vi "di_continuous_full.vi"() -> ()   [LabVIEW 2020]
uses:
  <vilib>/Waveform/DWDTOps.llb/DWDT Analog to Digital.vi
panel:
  out "DiFifoResidual":i32
  out "Rounds":i32
  in  "停止":bool
  out "error out":errorcluster caption="错误输出"
  out "数字波形图":digitalwaveform(graph)
  in  "SamplePeriod":u32=2000 caption="SamplePeriod (ns)"
  # "500k"
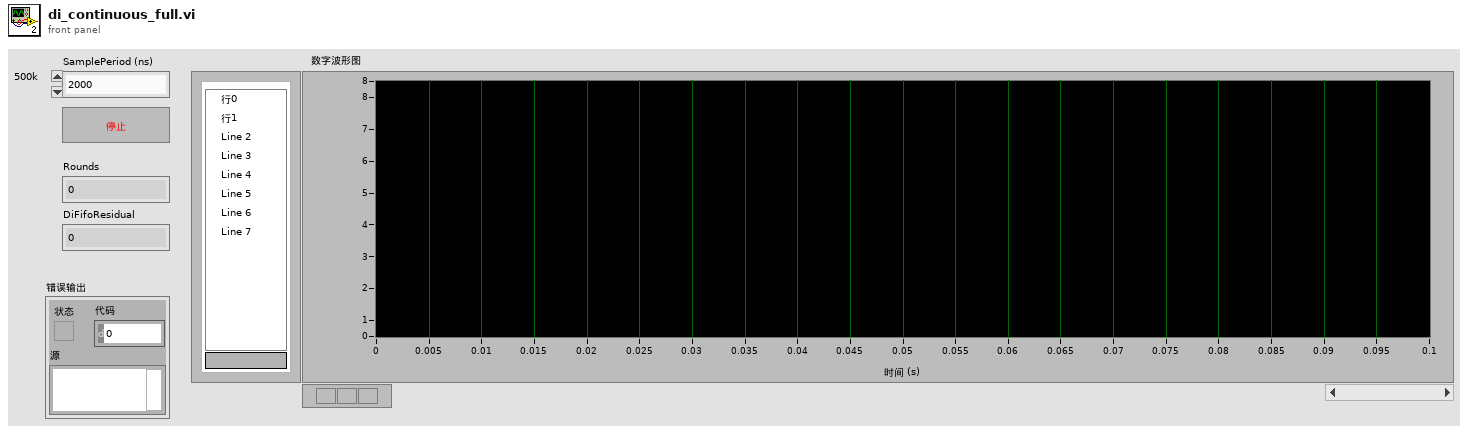
[diagram p1: front panel]
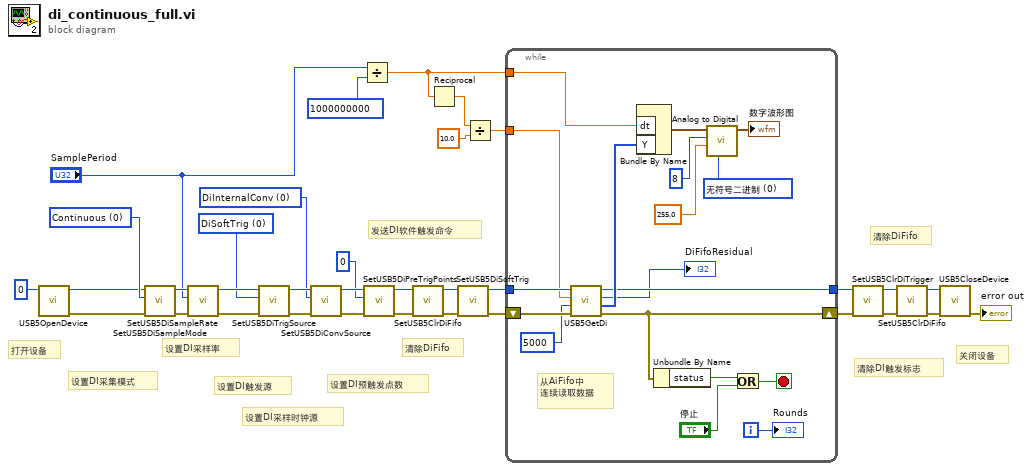
[diagram p0: block diagram]
diagram:
  w4 = u8 0 items=["DiInternalConv"=0, "ConvIn"=1, "AiConv"=2, "DoConv"=4, "Ao0Conv"=5, "Ao1Conv"=6, "Ao2Conv"=7, "Ao3Conv"=8] ("DiConvSource")
  w5 = u8 0 items=["DiSoftTrig"=0, "ExtTrigIn"=1, "Din0RisingEdge"=2, "Din1RisingEdge"=3, "Din2RisingEdge"=4, "Din3RisingEdge"=5, "WithAiTrig"=6, "WithDoTrig"=8, "WithAo0Trig"=9, "WithAo1Trig"=10, "WithAo2Trig"=11, "WithAo3Trig"=12, "GlobalSoftTrig"=255] ("DiTrigSource")
  w33 = u8 0 items=["Continuous", "OneShot"] ("DiSampleMode")
  # "关闭设备"
  # "清除DiFifo"
  # "清除DI触发标志"
  # "发送DI软件触发命令"
  # "清除DiFifo"
  # "设置DI预触发点数"
  # "设置DI采样时钟源"
  # "设置DI触发源"
  # "设置DI采样率"
  # "设置DI采集模式"
  # "打开设备"
  n1 = call "USB5OpenDevice.vi"("DevIndex"=0) -> ("error out"=w7:errorcluster, "DevIndex Out"=w8:i32)  [unwired: 9 in]
  n2 = call "SetUSB5DiSampleMode.vi"("错误输入（无错误）"=w7, "DiSampleMode"=w33, "DevIndex"=w8) -> ("错误输出"=w32:errorcluster, "DevIndex Out"=w31:i32)  [unwired: 7 in]
  n3 = call "SetUSB5DiSampleRate.vi"("错误输入（无错误）"=w32, "SamplePeriod(ns)"="SamplePeriod", "DevIndex"=w31) -> ("错误输出"=w18:errorcluster, "DevIndex Out"=w19:i32)  [unwired: 7 in]
  n4 = call "SetUSB5DiTrigSource.vi"("错误输入（无错误）"=w18, "DiTrigSource"=w5, "DevIndex"=w19) -> ("错误输出"=w16:errorcluster, "DevIndex Out"=w17:i32)  [unwired: 7 in]
  n5 = call "SetUSB5DiConvSource.vi"("错误输入（无错误）"=w16, "DiConvSource"=w4, "DevIndex"=w17) -> ("错误输出"=w14:errorcluster, "DevIndex Out"=w15:i32)  [unwired: 7 in]
  n6 = Divide(x="SamplePeriod", y=u32 1000000000) -> (x/y=w27:dbl)
  n7 = call "SetUSB5DiPreTrigPoints.vi"("错误输入（无错误）"=w14, "DiPreTrigPoints"=u32 0, "DevIndex"=w15) -> ("错误输出"=w10:errorcluster, "DevIndex Out"=w11:i32)  [unwired: 7 in]
  n8 = call "SetUSB5ClrDiFifo.vi"("错误输入（无错误）"=w10, "DevIndex"=w11) -> ("错误输出"=w13:errorcluster, "DevIndex Out"=w12:i32)  [unwired: 8 in]
  n9 = Reciprocal(x=w27) -> (1/x=w26:dbl)
  n10 = call "SetUSB5DiSoftTrig.vi"("错误输入（无错误）"=w13, "DevIndex"=w12) -> ("错误输出"=w29:errorcluster, "DevIndex Out"=w30:i32)  [unwired: 8 in]
  n11 = Divide(x=w26, y=10.0) -> (x/y=w25:dbl)
  n12 = while {
    tunnel: w27 -> [w45]
    shift-right: [w38] -> w20
    shift-left: w29 -> [w51]
    tunnel: w25 -> [w40]
    tunnel: w30 -> [w52]
    tunnel: [w39] -> w21
    i -> [w37]
    stop <- w41 stop-if-true
    w47 = u16 0 items=["无符号二进制", "二进制偏移量", "二进制补码"] ("data format (offset binary)")
    # "从AiFifo中\n连续读取数据"
    n13 = call "USB5GetDi.vi"("错误输入（无错误）"=w51, "TimeOut"=5000, "Points"=w40, "DevIndex"=w52) -> ("错误输出"=w38:errorcluster, "Di"=w44:u8[], "DiFifoUsed"=→"DiFifoResidual":i32, "DevIndex Out"=w39:i32)  [unwired: 4 in]
    n14 = Bundle By Name("dt"=w45, "Y"=w44) -> (w46:waveform(u8))  [unwired: 1 in]
    n15 = Unbundle By Name(w38) -> ("status"=w43:bool)
    n16 = call-poly <vilib>:"Analog to Digital.vi"("data format (offset binary)"=w47, "full-scale range (pk-pk)"=255.0, "resolution (16 bit)"=8, "analog waveform"=w46) -> ("digital waveform"=→"数字波形图":digitalwaveform)  [unwired: 4 in, 3 out]
    n17 = Or(x=w43, y="停止") -> (x .or. y?=w41:bool)
    "Rounds" <- w37
  }
  n18 = call "SetUSB5ClrDiTrigger.vi"("错误输入（无错误）"=w20, "DevIndex"=w21) -> ("错误输出"=w22:errorcluster, "DevIndex Out"=w23:i32)  [unwired: 8 in]
  n19 = call "SetUSB5ClrDiFifo.vi"("错误输入（无错误）"=w22, "DevIndex"=w23) -> ("错误输出"=w3:errorcluster, "DevIndex Out"=w2:i32)  [unwired: 8 in]
  n20 = call "USB5CloseDevice.vi"("错误输入（无错误）"=w3, "DevIndex"=w2) -> ("error out"=→"error out":errorcluster)  [unwired: 8 in, 1 out]
